vi "Temperature Sensing.vi"() -> ()   [LabVIEW 2020]
panel:
  out "Low Temp":bool
  out "Moderate Temp":bool
  out "High Temp":bool
  out "Meter":dbl(knob) scale=-20.0..50.0
  out "Temp":dbl
  in  "Temperature Sensor":dbl(slide) scale=-20.0..50.0
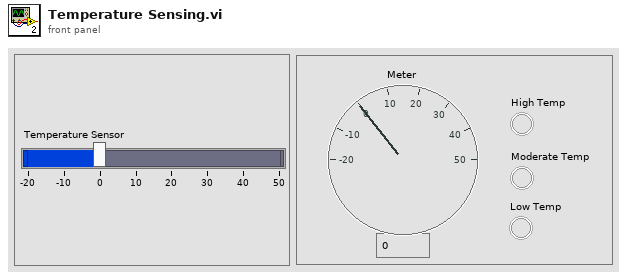
[diagram p1: front panel]
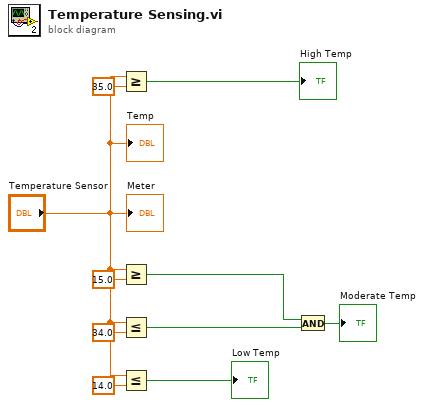
[diagram p0: block diagram]
diagram:
  n1 = Greater Or Equal?(x="Temperature Sensor", y=35.0) -> (x >= y?=→"High Temp":bool)
  n2 = Greater Or Equal?(x="Temperature Sensor", y=15.0) -> (x >= y?=w6:bool)
  n3 = Less Or Equal?(x="Temperature Sensor", y=34.0) -> (x <= y?=w5:bool)
  n4 = Less Or Equal?(x="Temperature Sensor", y=14.0) -> (x <= y?=→"Low Temp":bool)
  n5 = And(x=w6, y=w5) -> (x .and. y?=→"Moderate Temp":bool)
  "Temp" <- "Temperature Sensor"
  "Meter" <- "Temperature Sensor"
